vi "Graph Set Cursor Mode.vi"(8 "error in":errorcluster, 10 "Cursor Mode":enum32{"Free-Drag", "Single-Plot", "Multi-Plot"}(ring), 11 "Graph Refs in":refnum<vi>[](array[refnum])) -> (0 "error out":errorcluster, 3 "Graph Refs out":refnum<vi>[](array[refnum]))   [LabVIEW 2023, in "FPT Framework UI.lvlib"]
doc: "Use this VI to update the cursor type on the selected graphs."
uses:
  FPT Framework UI.lvlib
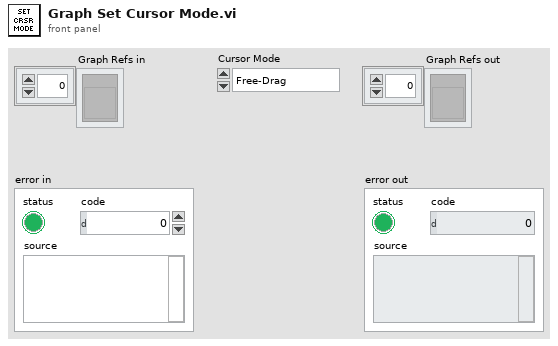
[diagram p1: front panel]
types:
  T1 = typedef "LVCursorListTypeDef.ctl" = cluster{"Name":string, "Color":u32, "Style":u8, "Point Style":u8, "Name Visible":bool, "Allow Drag":bool, "Cursor Mode":u32, "Plot":i32, "Index":i32, "Position":cluster{"X":dbl, "Y":dbl}, "X Scale":u32, "Y Scale":u32, "Watch Plots":i32[], "Watch All Plots":bool, "Plot Area":i32, "Label Offset":cluster{"X":dbl, "Y":dbl}}[]
  T2 = cluster{"Name":string, "Color":u32, "Style":u8, "Point Style":u8, "Name Visible":bool, "Allow Drag":bool, "Cursor Mode":u32, "Plot":i32, "Index":i32, "Position":cluster{"X":dbl, "Y":dbl}, "X Scale":u32, "Y Scale":u32, "Watch Plots":i32[], "Watch All Plots":bool, "Plot Area":i32, "Label Offset":cluster{"X":dbl, "Y":dbl}}
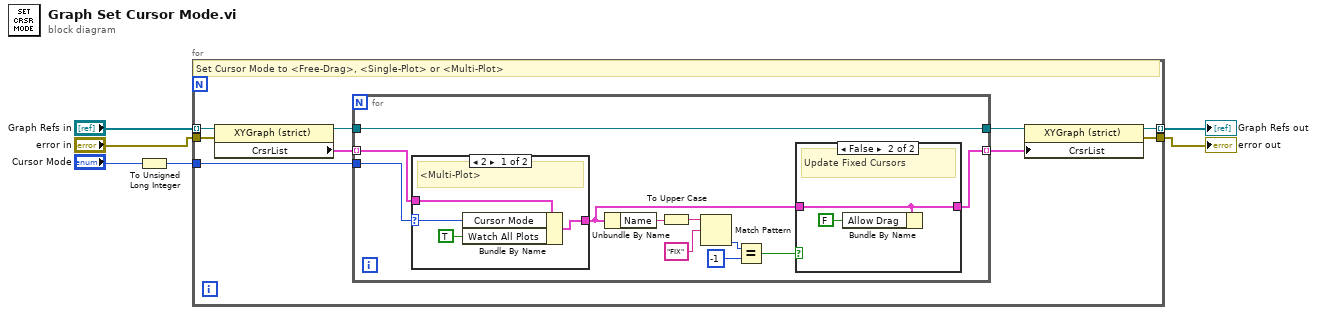
[diagram p0: block diagram]
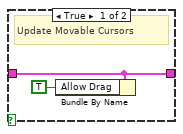
[diagram p2: hidden frame]
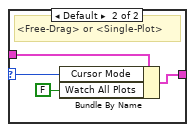
[diagram p3: hidden frame]
diagram:
  n1 = To Unsigned Long Integer(number="Cursor Mode") -> (unsigned 32bit integer=w1:u32)
  n2 = for {
    tunnel: "Graph Refs in" -> [w15] mode=indexing
    tunnel: [w10] -> w3
    tunnel: "error in" -> [w9]
    tunnel: [w8] -> w6 mode=indexing
    tunnel: w1 -> [w7]
    # "Set Cursor Mode to <Free-Drag>, <Single-Plot> or <Multi-Plot>"
    n3 = property class="XYGraph (strict)"(reference=w15, error in=w9) -> (reference out=w14:refnum<vi>, "CrsrList"=w13:T1)  [unwired: 1 out]
    n4 = for {
      tunnel: w14 -> [w25]
      tunnel: w13 -> [w26] mode=indexing
      tunnel: [w16] -> w12 mode=indexing
      tunnel: [w25] -> w11
      tunnel: w7 -> [w24]
      n5 = case shown="2" w24 {
        selector: w24 -> [w32 w36]
        tunnel: w26 -> [w34 w38]
        tunnel: [w33 w37] -> w17
        frame 2 {
          # "<Multi-Plot>"
          n6 = Bundle By Name(cluster=w34, "Cursor Mode"=w32, "Watch All Plots"=TRUE) -> (w33:T2)
        }
        frame Default {
          # "<Free-Drag> or <Single-Plot>"
          n7 = Bundle By Name(cluster=w38, "Cursor Mode"=w36, "Watch All Plots"=FALSE) -> (w37:T2)
        }
      }
      n8 = Unbundle By Name(w17) -> ("Name"=w19:string)
      n9 = To Upper Case(1:w19) -> (0:w22:string)
      n10 = Match Pattern(string=w22, regular expression="FIX") -> (offset past match=w21:i32)  [unwired: 1 in, 3 out]
      n11 = Equal?(x=w21, y=-1) -> (x = y?=w18:bool)
      n12 = case shown="False" w18 {
        tunnel: w17 -> [w27 w29]
        tunnel: [w27 w29] -> w16
        frame True {
          # "Update Movable Cursors"
          n13 = Bundle By Name(cluster=w27, "Allow Drag"=TRUE) -> ()  [unwired: 1 out]
        }
        frame False {
          # "Update Fixed Cursors"
          n14 = Bundle By Name(cluster=w29, "Allow Drag"=FALSE) -> ()  [unwired: 1 out]
        }
      }
    }
    n15 = property class="XYGraph (strict)"(reference=w11, "CrsrList"=w12) -> (reference out=w8:refnum<vi>, error out=w10:errorcluster)  [unwired: 1 in]
  }
  "Graph Refs out" <- w6
  "error out" <- w3
